vi "Base64Encoder.vi"(11 "String In":string) -> (2 "Base64ByteArray":u8[](array[numeric]) format="%b", 3 "String Out":string)   [LabVIEW 2014]
doc: "Encode a binary string as a base64 encoded string"
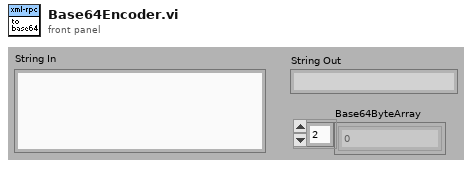
[diagram p1: front panel]
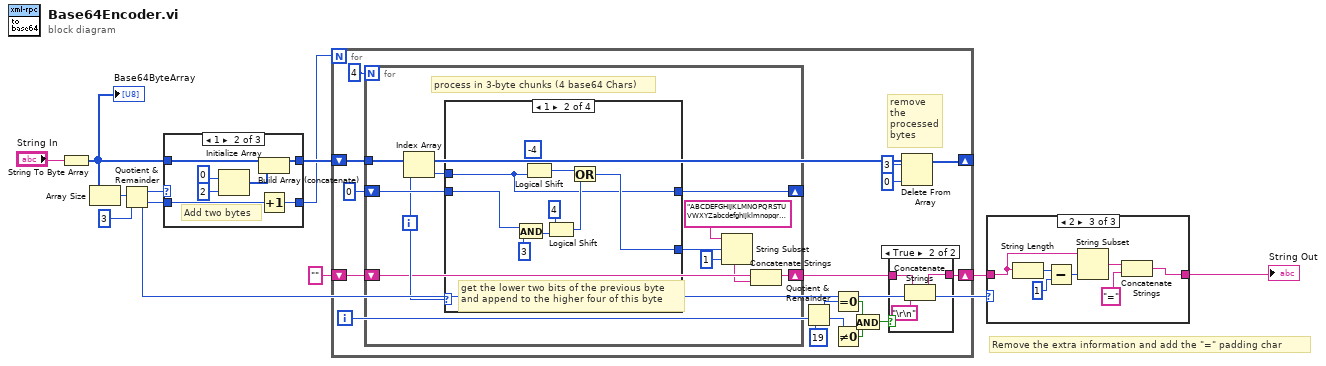
[diagram p0: block diagram]
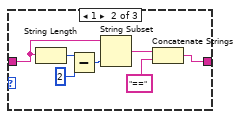
[diagram p3: hidden frame]
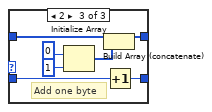
[diagram p5: hidden frame]
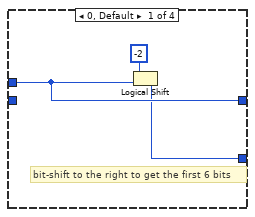
[diagram p7: hidden frame]
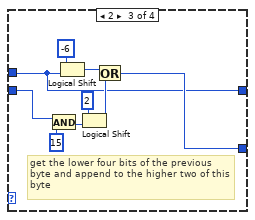
[diagram p8: hidden frame]
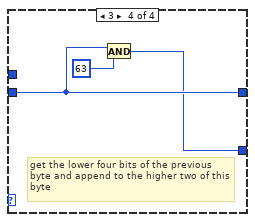
[diagram p9: hidden frame]
diagram:
  # "Remove the extra information and add the \"=\" padding char"
  n1 = String To Byte Array(string="String In") -> (unsigned byte array=w5:u8[])
  "Base64ByteArray" <- w5
  n2 = Array Size(array=w5) -> (size(s)=w10:i32)
  n3 = Quotient & Remainder(x=w10, y=3) -> (x-y*floor(x/y)=w3:i32, floor(x/y)=w8:i32)
  n4 = case shown="1" w3 {
    tunnel: w5 -> [w13 w20 w27]
    tunnel: [w13 w19 w26] -> w9
    tunnel: w8 -> [w12 w15 w22]
    tunnel: [w12 w14 w21] -> w7
    frame 0, Default {
    }
    frame 1 {
      # "Add two bytes"
      n5 = Initialize Array(u8 0, 2 ("dimension size")) -> (w16:u8[])
      n6 = Build Array (concatenate)(w20, w16) -> (w19:u8[])
      n7 = Increment(x=w15) -> (x+1=w14:i32)
    }
    frame 2 {
      # "Add one byte"
      n8 = Initialize Array(u8 0, 1 ("dimension size")) -> (w23:u8[])
      n9 = Build Array (concatenate)(w27, w23) -> (w26:u8[])
      n10 = Increment(x=w22) -> (x+1=w21:i32)
    }
  }
  n11 = for {
    N: w7 -> [_]
    shift-right: [w37] -> _
    shift-left: w9 -> [w40]
    shift-right: [w34] -> w4
    shift-left: "" -> [w36]
    i -> [w28]
    # "remove the processed bytes"
    n12 = for {
      N: 4 -> [_]
      tunnel: w40 -> [w57]
      shift-right: [w55] -> _
      shift-left: u8 0 -> [w54]
      shift-right: [w47] -> w35
      shift-left: w36 -> [w49]
      i -> [w53]
      # "process in 3-byte chunks (4 base64 Chars)"
      n13 = Index Array(array=w57, index=w53) -> (element=w56:u8)
      n14 = case shown="1" w53 {
        tunnel: w56 -> [w59 w61 w70 _]
        tunnel: [w59 w61 w70 w80] -> w55
        tunnel: [w58 w62 w71 w79] -> w52
        tunnel: w54 -> [_ w69 w78 w80]
        frame 0, Default {
          # "bit-shift to the right to get the first 6 bits"
          n15 = Logical Shift(y=i8 -2, x=w59) -> (x << y=w58:u8)
        }
        frame 1 {
          # "get the lower two bits of the previous byte\nand append to the higher four of this byte"
          n16 = And(x=w69, y=u8 3) -> (x .and. y?=w67:u8)
          n17 = Logical Shift(y=i8 -4, x=w61) -> (x << y=w64:u8)
          n18 = Logical Shift(y=u8 4, x=w67) -> (x << y=w63:u8)
          n19 = Or(x=w64, y=w63) -> (x .or. y?=w62:u8)
        }
        frame 2 {
          # "get the lower four bits of the previous byte and append to the higher two of this byte"
          n20 = And(x=w78, y=u8 15) -> (x .and. y?=w76:u8)
          n21 = Logical Shift(y=i8 -6, x=w70) -> (x << y=w73:u8)
          n22 = Logical Shift(y=u8 2, x=w76) -> (x << y=w72:u8)
          n23 = Or(x=w73, y=w72) -> (x .or. y?=w71:u8)
        }
        frame 3 {
          # "get the lower four bits of the previous byte and append to the higher two of this byte"
          n24 = And(x=w80, y=u8 63) -> (x .and. y?=w79:u8)
        }
      }
      n25 = String Subset(string="ABCDEFGHIJKLMNOPQRSTUVWXYZabcdefghijklmnopqrstuvwxyz0123456789+/", offset (0)=w52, length (rest)=1 ("length (rest)")) -> (substring=w48:string)
      n26 = Concatenate Strings(w49, w48) -> (w47:string)
    }
    n27 = Quotient & Remainder(x=w28, y=19) -> (x-y*floor(x/y)=w30:i32)  [unwired: 1 out]
    n28 = Equal To 0?(x=w30) -> (x = 0?=w29:bool)
    n29 = Not Equal To 0?(x=w28) -> (x != 0?=w31:bool)
    n30 = And(x=w29, y=w31) -> (x .and. y?=w33:bool)
    n31 = case shown="True" w33 {
      tunnel: [w43 w46] -> w34
      tunnel: w35 -> [w43 w45]
      frame False {
      }
      frame True {
        n32 = Concatenate Strings(w45, "\r\n") -> (w46:string)
      }
    }
    n33 = Delete From Array(array=w40, length=3, index=0) -> (array with subset deleted=w37:u8[])  [unwired: 1 out]
  }
  n34 = case shown="2" w3 {
    tunnel: w4 -> [w82 w89 w96]
    tunnel: [w82 w85 w92] -> w2
    frame 0, Default {
    }
    frame 1 {
      n35 = String Length(string=w89) -> (length=w87:i32)
      n36 = Subtract(x=w87, y=2) -> (x-y=w88:i32)
      n37 = String Subset(string=w89, length (rest)=w88) -> (substring=w86:string)  [unwired: 1 in]
      n38 = Concatenate Strings(w86, "==" ("Substring")) -> (w85:string)
    }
    frame 2 {
      n39 = String Length(string=w96) -> (length=w94:i32)
      n40 = Subtract(x=w94, y=1) -> (x-y=w95:i32)
      n41 = String Subset(string=w96, length (rest)=w95) -> (substring=w93:string)  [unwired: 1 in]
      n42 = Concatenate Strings(w93, "=" ("Substring")) -> (w92:string)
    }
  }
  "String Out" <- w2
